vi "chaos crest cu cmd.vi"(7 "args":string, 9 "cmd":string, 10 "cuname":string, 11 "h":u32) -> (2 "function return":i32, 3 "h out":u32)   [LabVIEW 2014, in "libcommon-crest.lvlib"]
doc: "int chaos_crest_cu_cmd(chaos_crest_handle_t h,const char*cuname,const char*cmd,const char* args);"
uses:
  libcommon-crest.lvlib
  chaos-i686-dynamic-release/lib/libcommon-crest.so
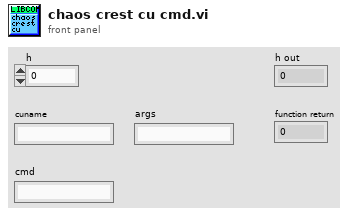
[diagram p1: front panel]
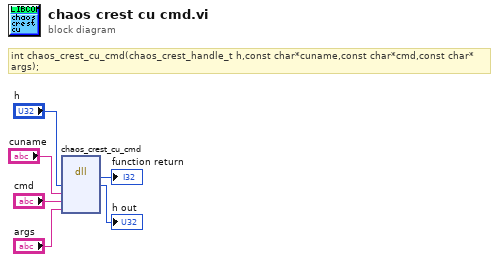
[diagram p0: block diagram]
diagram:
  # "int chaos_crest_cu_cmd(chaos_crest_handle_t h,const char*cuname,const char*cmd,const char* args);"
  n1 = dll-call lib="home/chaos/chaos_bundle/chaos-i686-dynamic-release/lib/libcommon-crest.*" fn="chaos_crest_cu_cmd"("h"="h", "cuname"="cuname", "cmd"="cmd", "args"="args") -> (→"function return":i32, "h"=→"h out":u32)  [unwired: 6 in, 2 out]
